vi "load_saved_scan_settings.vi"(8 "error in (no error)":errorcluster, 11 "User name":string) -> (0 "error out":errorcluster, 1 "Scan settings array":T1[](array[typedef]) {"Electrode configuration" items=["2-wire", "4-wire"]; "Logarithmic sweep" items=["False", "True"]; "Repeat scans" items=["True", "False"]; "No. of repeat scans" min=1.0 step=1.0; "Stabilisation mode" items=["V", "I"]; "Dual sweep" items=["True", "False"]; "Measurement delay (ms)" min=10.0}, 3 "Scan settings name array":string[](array[string]), 4 "Settings folder path":path)   [LabVIEW 2016]
uses:
  TypeDefs/settings.ctl
  <vilib>/Utility/file.llb/Read Delimited Spreadsheet (string).vi
  <vilib>/Utility/file.llb/Write Delimited Spreadsheet (string).vi
panel:
  in  "Deafult_std":string[](array[string])=["1", "0", "-1.4", "0.1", "0.02", "10", "1", "0", "5", "0", "-1.4", "5", "0", "0", "0", "-1.4", "0.1", "0.1", "0", "1", "0", "1", "0.7", "30", "0", "0", "0", "0", "0", "0", "0", "310", "900", "5", "200", "2", "0", "120", "4", "0.25", "2", "1", "1", "1", "0", "1", "0", "1", "0"]
  in  "Deafult_inv":string[](array[string])=["1", "0", "-0.1", "1.4", "0.02", "10", "1", "1", "0", "0", "1.4", "5", "0", "0", "1", "-0.1", "1.4", "0.1", "0", "1", "1", "1", "0.7", "30", "0", "0", "0", "0", "0", "0", "0", "310", "900", "5", "200", "2", "0", "120", "4", "0.25", "0", "1", "1", "1", "0", "1", "0", "1", "0"]
  out "String":string
  out "all rows":string[][](array[string])
  in  "Scan settings":T1={"Start voltage (V)"=0.0, "End voltage (V)"=1.4, "Number of steps"=0, "Measurement delay (ms)"=1.4, "Dual sweep"=0, "Stabilisation time (s)"=10.0, "Stabilisation mode"=0, "Stabilisation value (V or A) "=0.0, "No. of repeat scans"=0.0, "Repeat scans"=0, "Logarithmic sweep"=0, "Electrode configuration"=0} {"Electrode configuration" items=["2-wire", "4-wire"]; "Logarithmic sweep" items=["False", "True"]; "Repeat scans" items=["True", "False"]; "No. of repeat scans" min=1.0 step=1.0; "Stabilisation mode" items=["V", "I"]; "Dual sweep" items=["True", "False"]; "Measurement delay (ms)" min=10.0}
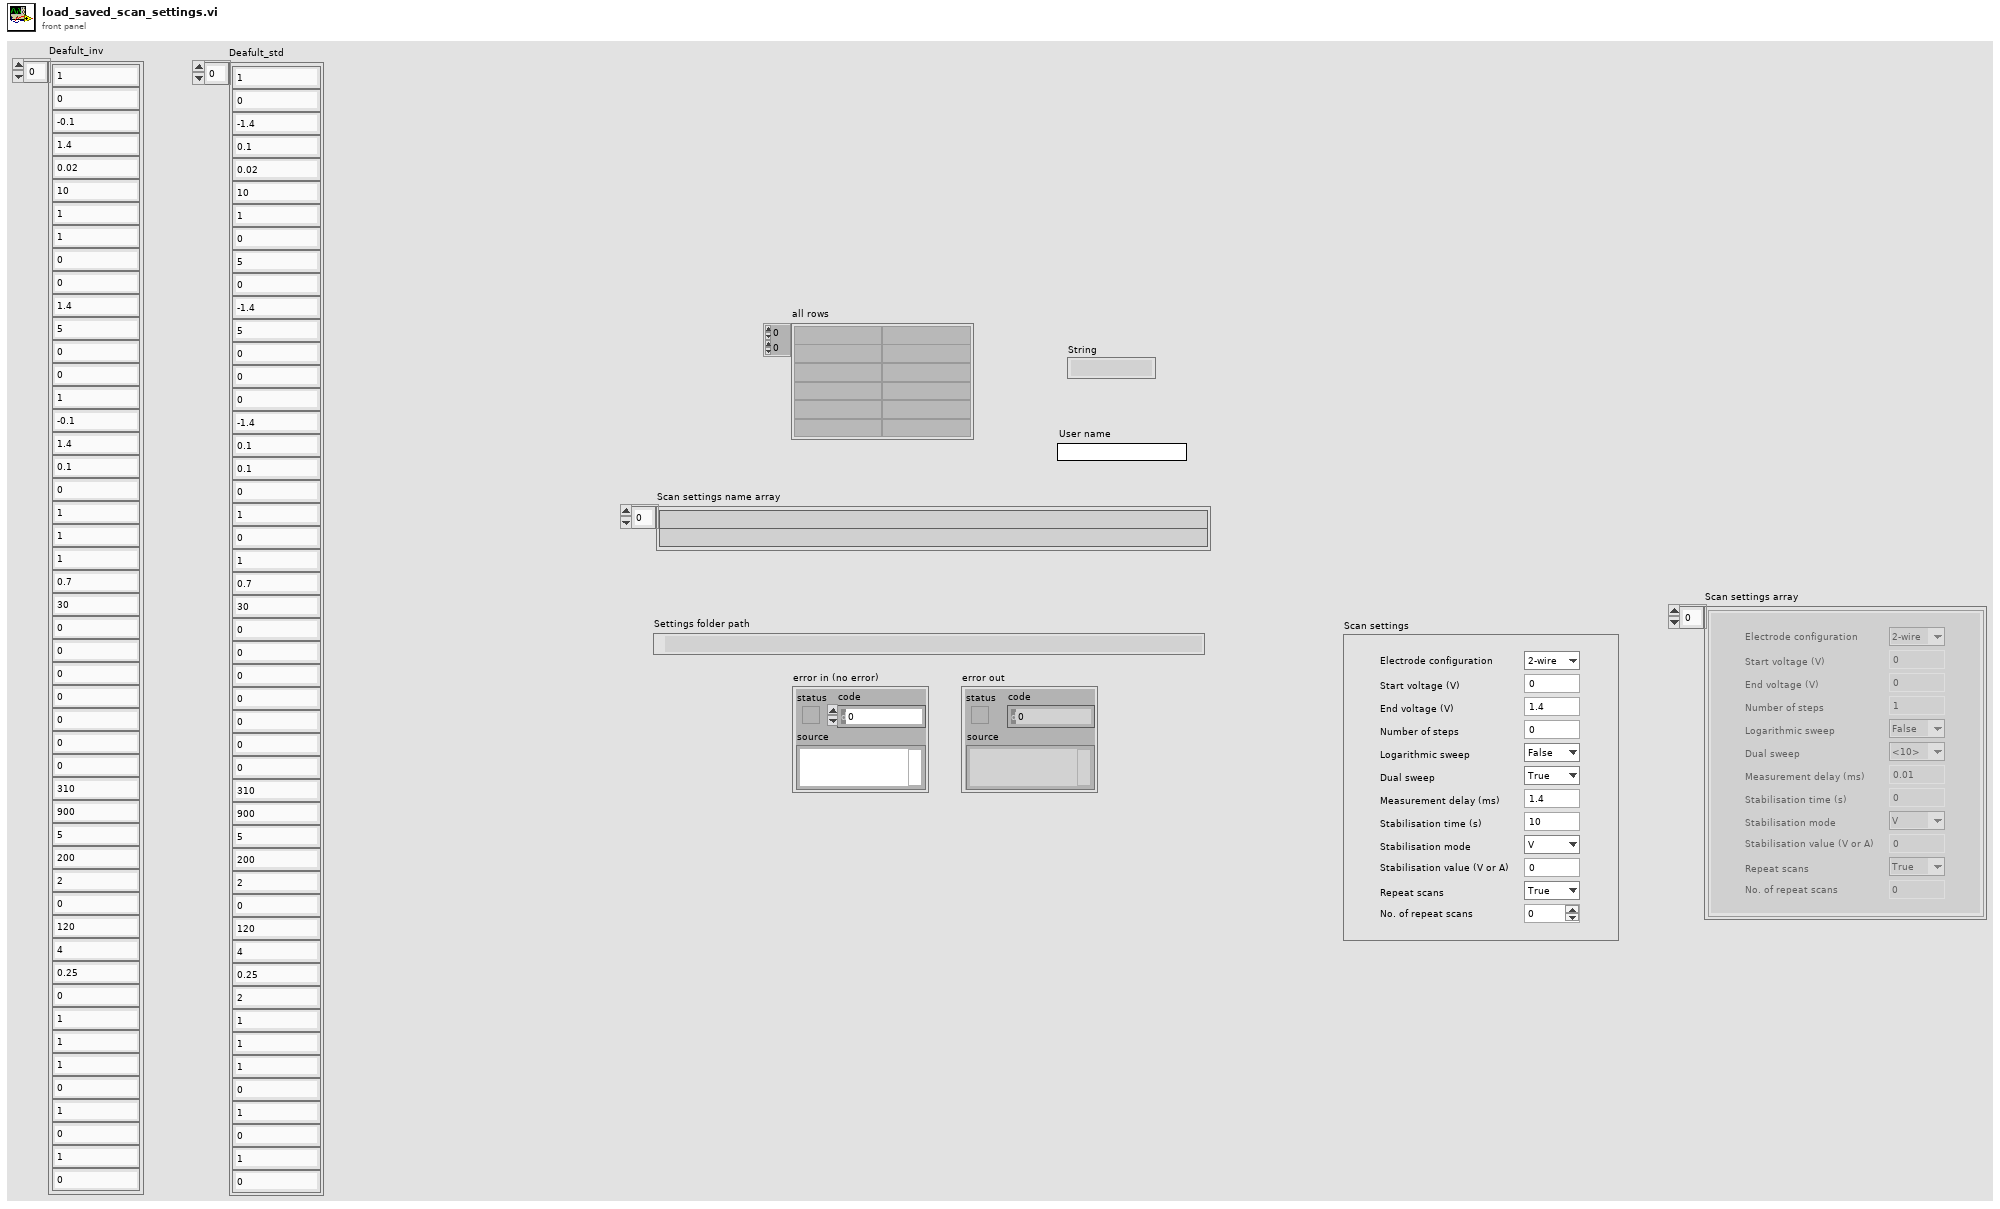
[diagram p1: front panel]
types:
  T1 = typedef "settings.ctl" = cluster{"Start voltage (V)":dbl, "End voltage (V)":dbl, "Number of steps":u32, "Measurement delay (ms)":dbl, "Dual sweep":u16, "Stabilisation time (s)":dbl, "Stabilisation mode":u16, "Stabilisation value (V or A) ":dbl, "No. of repeat scans":dbl, "Repeat scans":u16, "Logarithmic sweep":u16, "Electrode configuration":u16}
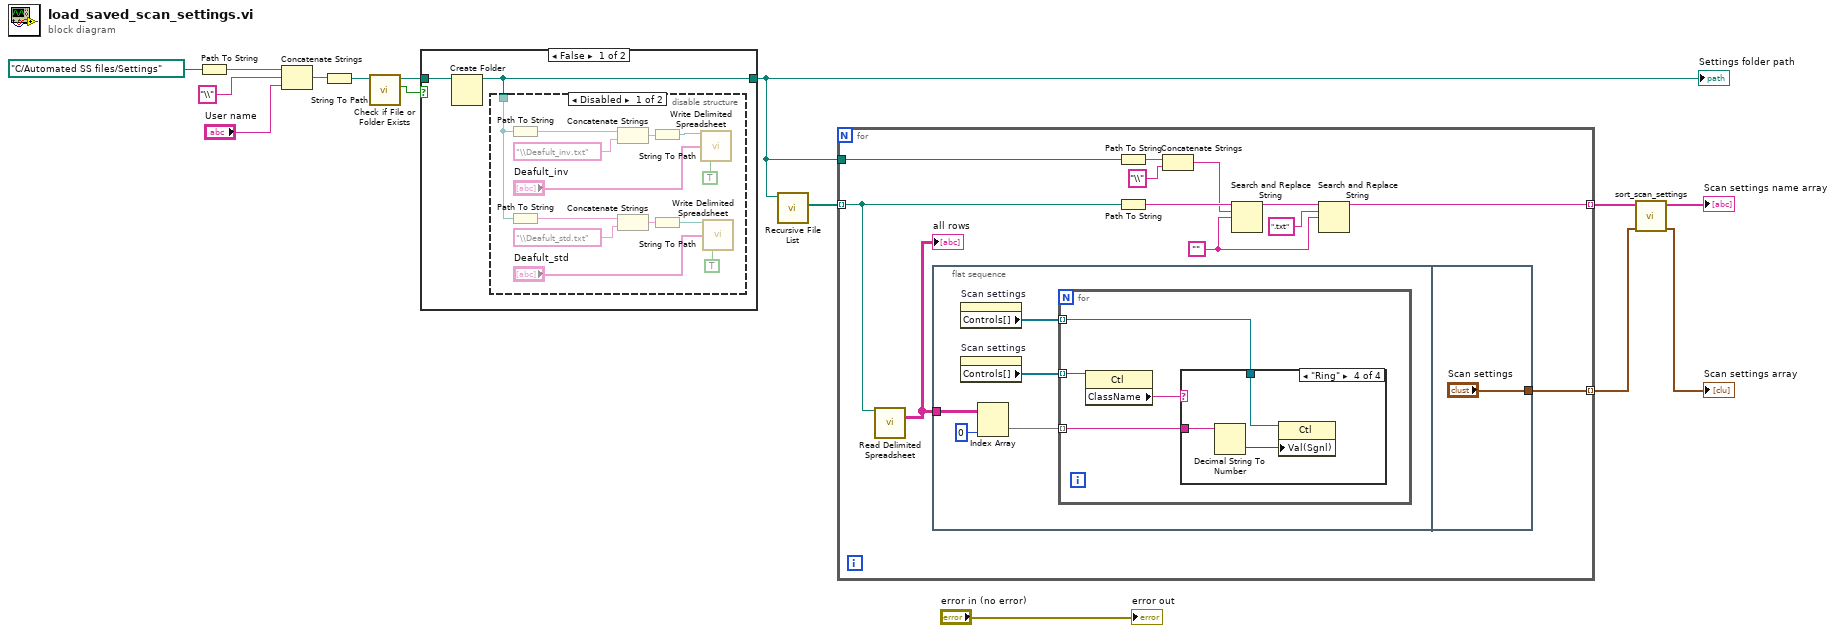
[diagram p0: block diagram]
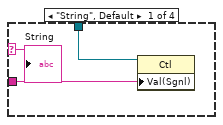
[diagram p4: hidden frame]
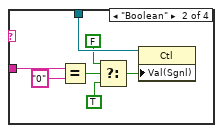
[diagram p5: hidden frame]
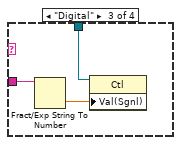
[diagram p6: hidden frame]
diagram:
  n1 = Path To String(path=path "C:/Automated SS files/Settings") -> (string=w9:string)
  n2 = Concatenate Strings(w9, "\\", "User name") -> (w1:string)
  n3 = String To Path(string=w1) -> (path=w4:path)
  n4 = call <vilib>:"Check if File or Folder Exists.vi"("path"=w4) -> ("file or folder exists?"=w6:bool, "dup path"=w5:path)  [unwired: 8 in, 1 out]
  n5 = case shown="False" w6 {
    tunnel: w5 -> [w17 w31]
    tunnel: [w16 w31] -> w2
    frame False {
      n6 = Create Folder(path (use dialog)=w17) -> (created path=w16:path)  [unwired: 2 in, 2 out]
      n7 = disable-structure shown="Disabled" {
        disable-tunnel: w16 -> [w24 _]
        frame Disabled {
          n8 = Path To String(path=w24) -> (string=w29:string)
          n9 = Path To String(path=w24) -> (string=w25:string)
          n10 = Concatenate Strings(w29, "\\Deafult_inv.txt") -> (w28:string)
          n11 = Concatenate Strings(w25, "\\Deafult_std.txt") -> (w22:string)
          n12 = String To Path(string=w28) -> (path=w27:path)
          n13 = String To Path(string=w22) -> (path=w23:path)
          n14 = call-poly <vilib>:"Write Delimited Spreadsheet.vi"("file path (dialog if empty)"=w27, "1D data"="Deafult_inv", "transpose? (no:F)"=TRUE) -> ()  [unwired: 11 in, 2 out]
          n15 = call-poly <vilib>:"Write Delimited Spreadsheet.vi"("file path (dialog if empty)"=w23, "1D data"="Deafult_std", "transpose? (no:F)"=TRUE) -> ()  [unwired: 11 in, 2 out]
        }
        frame Enabled {
        }
      }
    }
    frame True {
    }
  }
  "Settings folder path" <- w2
  n16 = call <vilib>:"Recursive File List.vi"("Folder Path"=w2) -> ("All Files in Dir"=w15:path[])  [unwired: 6 in, 4 out]
  n17 = for {
    tunnel: w15 -> [w34] mode=indexing
    tunnel: w2 -> [w36]
    tunnel: [w35] -> w13 mode=indexing
    tunnel: [w33] -> w11 mode=indexing
    w41 = ""
    n18 = call-poly <vilib>:"Read Delimited Spreadsheet.vi"("file path (dialog if empty)"=w34) -> ("all rows"=w32:string[][])  [unwired: 9 in, 5 out]
    "all rows" <- w32
    n19 = flat-sequence {
      tunnel: w32 -> [w46]
      tunnel: ["Scan settings"] -> w33
      frame #0 {
        n20 = property on="Scan settings" class="Clust (strict)"() -> ("Controls[]"=w47:refnum<vi>[])  [unwired: 2 in, 2 out]
        n21 = property on="Scan settings" class="Clust (strict)"() -> ("Controls[]"=w48:refnum<vi>[])  [unwired: 2 in, 2 out]
        n22 = Index Array(array=w46, index (col)=0 ("disabled index (col)")) -> (element=w44:string[])  [unwired: 1 in]
        n23 = for {
          tunnel: w48 -> [w52] mode=indexing
          tunnel: w47 -> [w50] mode=indexing
          tunnel: w44 -> [w49] mode=indexing
          n24 = property class="Ctl"(reference=w52) -> ("ClassName"=w51:string)  [unwired: 1 in, 2 out]
          n25 = case shown="\"Ring\"" w51 {
            selector: w51 -> [w53 _ _ _]
            tunnel: w50 -> [w55 w62 w65 w67]
            tunnel: w49 -> [w54 w61 w64 w68]
            frame "String", Default {
              n26 = property class="Ctl"(reference=w55, "Val(Sgnl)"=w54) -> ()  [unwired: 1 in, 2 out]
              "String" <- w53
            }
            frame "Boolean" {
              n27 = Equal?(x=w61, y="0") -> (x = y?=w59:bool)
              n28 = Select(t=FALSE, s=w59, f=TRUE) -> (s? t:f=w56:bool)
              n29 = property class="Ctl"(reference=w62, "Val(Sgnl)"=w56) -> ()  [unwired: 1 in, 2 out]
            }
            frame "Digital" {
              n30 = Fract/Exp String To Number(string=w64) -> (number=w63:dbl)  [unwired: 3 in, 1 out]
              n31 = property class="Ctl"(reference=w65, "Val(Sgnl)"=w63) -> ()  [unwired: 1 in, 2 out]
            }
            frame "Ring" {
              n32 = Decimal String To Number(string=w68) -> (number=w66:i32)  [unwired: 2 in, 1 out]
              n33 = property class="Ctl"(reference=w67, "Val(Sgnl)"=w66) -> ()  [unwired: 1 in, 2 out]
            }
          }
        }
      }
      frame #1 {
      }
    }
    n34 = Path To String(path=w36) -> (string=w39:string)
    n35 = Path To String(path=w34) -> (string=w42:string)
    n36 = Concatenate Strings(w39, "\\") -> (w37:string)
    n37 = Search and Replace String(input string=w42, search string=w37, replace string=w41) -> (result string=w40:string)  [unwired: 5 in, 3 out]
    n38 = Search and Replace String(input string=w40, search string=".txt", replace string=w41) -> (result string=w35:string)  [unwired: 5 in, 3 out]
  }
  n39 = call "sort_scan_settings.vi"("Scan settings array"=w11, "Setting name array"=w13) -> ("Sorted settings array"=→"Scan settings array":T1[], "Sorted name array"=→"Scan settings name array":string[])  [unwired: 7 in]
  "error out" <- "error in (no error)"
